vi "Release-refs.vi"(8 "error in (no error)":errorcluster, 11 "UI ref. in":refnum<data-value>) -> (0 "error out":errorcluster, 3 "UI ref.":refnum<data-value>)   [LabVIEW 2013, in "CameraVision.lvlib" / "CV-UI.lvclass"]
uses:
  CV-UI.lvclass
  CV-UI.lvclass/CV-UI.ctl
  Read Control refs.vi
  Read Display refs.vi
  Read Parameter refs.vi
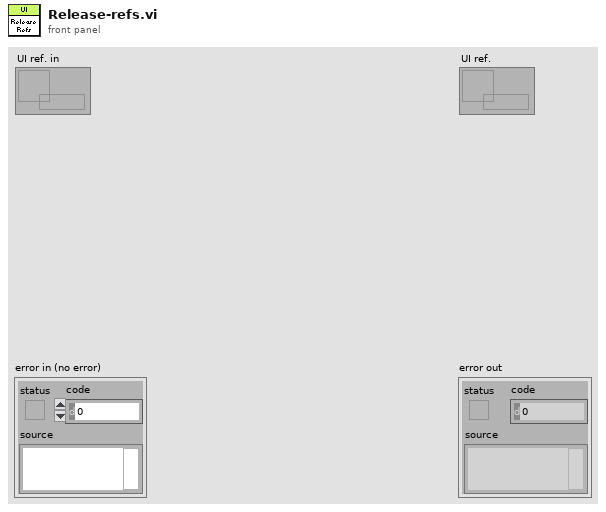
[diagram p1: front panel]
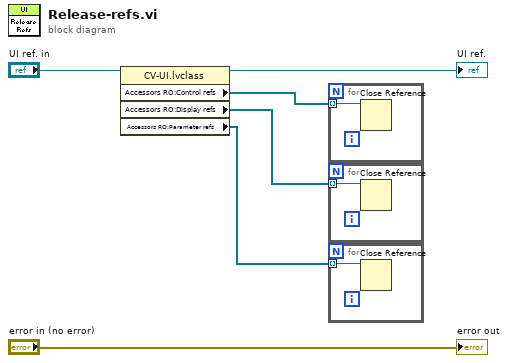
[diagram p0: block diagram]
diagram:
  n1 = property class="CV-UI.lvclass"(reference="UI ref. in") -> (reference out=→"UI ref.":refnum<data-value>, "Accessors RO:Control refs"=w3:refnum<vi>[], "Accessors RO:Display refs"=w2:refnum<vi>[], "Accessors RO:Parameter refs"=w1:refnum<vi>[])  [unwired: 1 in, 1 out]
  n2 = for {
    tunnel: w3 -> [w7] mode=indexing
    n3 = Close Reference(reference=w7) -> ()  [unwired: 1 in, 1 out]
  }
  n4 = for {
    tunnel: w2 -> [w8] mode=indexing
    n5 = Close Reference(reference=w8) -> ()  [unwired: 1 in, 1 out]
  }
  n6 = for {
    tunnel: w1 -> [w9] mode=indexing
    n7 = Close Reference(reference=w9) -> ()  [unwired: 1 in, 1 out]
  }
  "error out" <- "error in (no error)"
